vi "ParseDataNoPWM.vi"(1 "input string":string) -> (0 "output cluster":T1)   [LabVIEW 2023]
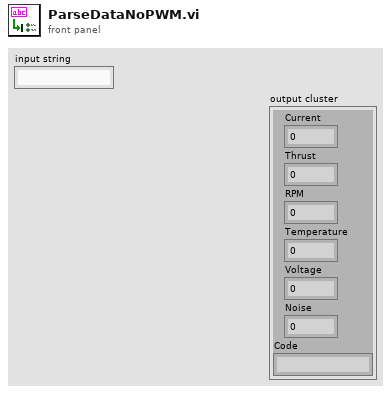
[diagram p1: front panel]
types:
  T1 = cluster{"Current":dbl, "Thrust":dbl, "RPM":dbl, "Temperature":dbl, "Voltage":dbl, "Noise":dbl, "Code":string}
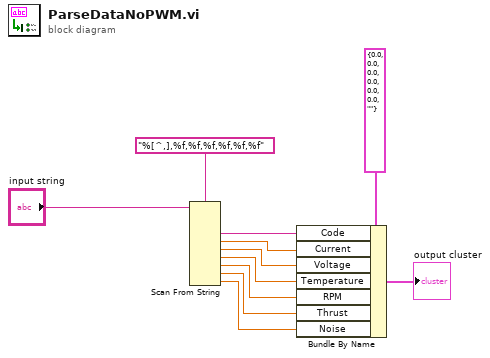
[diagram p0: block diagram]
diagram:
  n1 = Scan From String(format string="%[^,],%f,%f,%f,%f,%f,%f", input string="input string") -> (output 1=w5:string, output 2=w6:dbl, output 3=w7:dbl, output 4=w8:dbl, output 5=w9:dbl, output 6=w10:dbl, output 7=w11:dbl)  [unwired: 9 in, 3 out]
  n2 = Bundle By Name(cluster=T1 {"Current"=0.0, "Thrust"=0.0, "RPM"=0.0, "Temperature"=0.0, "Voltage"=0.0, "Noise"=0.0, "Code"=""} ("Data"), "Code"=w5, "Current"=w6, "Voltage"=w7, "Temperature"=w8, "RPM"=w9, "Thrust"=w10, "Noise"=w11) -> (→"output cluster":T1)
